vi "Get_file_list_table.vi"(10 "Filter pattern":string="*.xls", 11 "file path (dialog if empty)":path=path "C:/RIMAS/Temperature-logs") -> (0 "Files names":string[][](array[string]), 1 "selected path":path, 2 "Multicolumn Listbox":i32[](listbox), 3 "All Files in Dir":path[](array[path]))   [LabVIEW 2012]
panel:
  out "Array 2":dbl[](array[numeric])
  out "Justify arr":enum16{"Left", "Center", "Right"}[](array[ring])
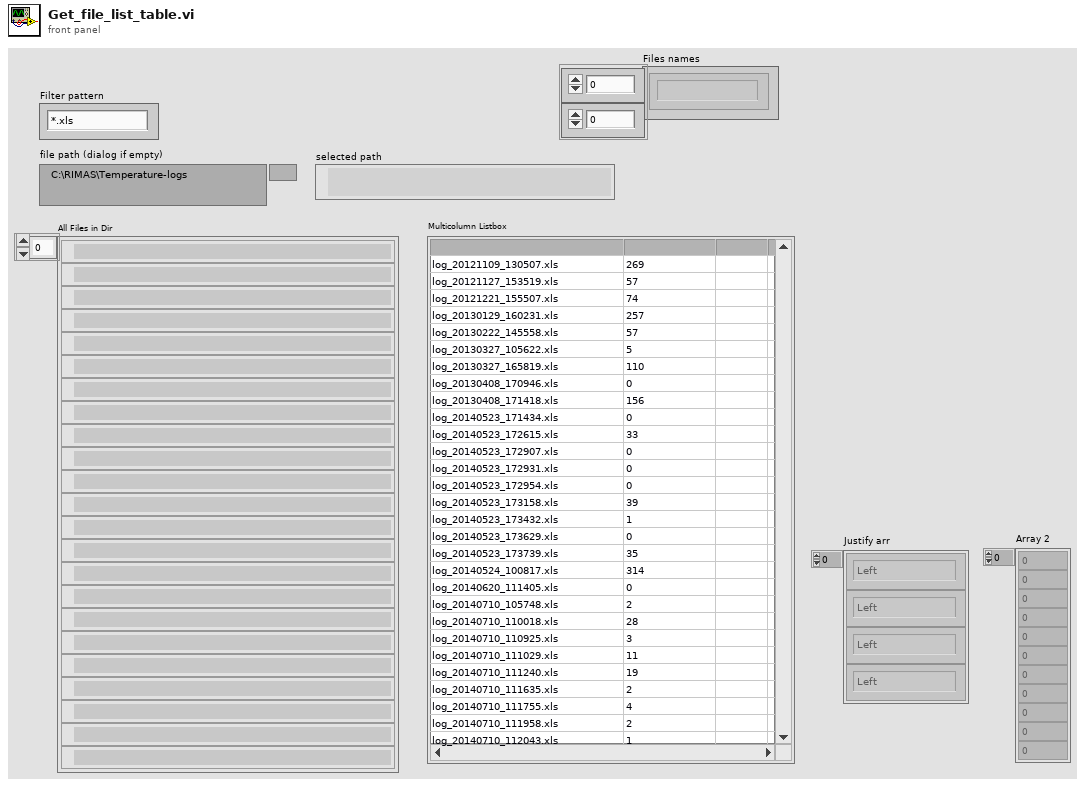
[diagram p1: front panel]
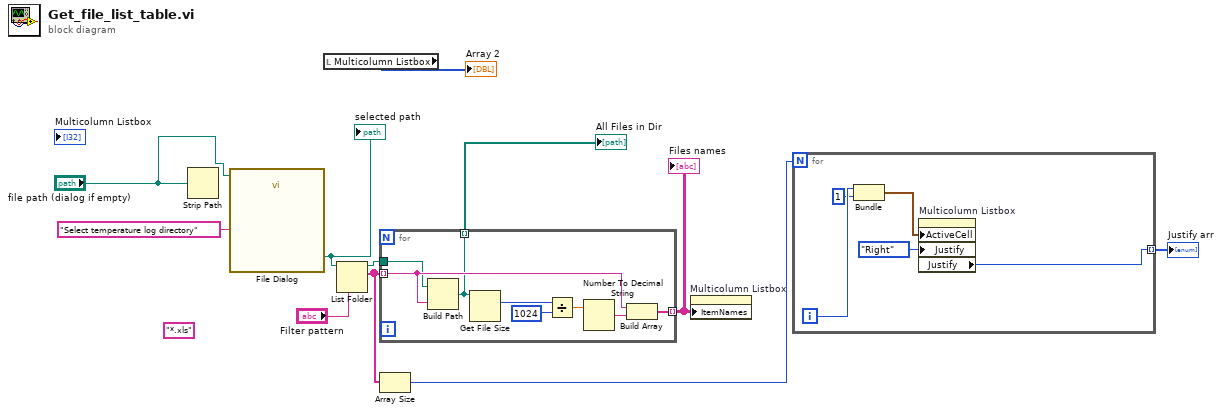
[diagram p0: block diagram]
diagram:
  (unwired) "*.xls" ("pattern (all files)")
  n1 = Strip Path(path="file path (dialog if empty)") -> ()  [unwired: 2 out]
  n2 = call "File Dialog"("start path"="file path (dialog if empty)", "prompt"="Select temperature log directory") -> ("selected path"=w11:path)  [unwired: 10 in, 3 out]
  "selected path" <- w11
  n3 = local read "Multicolumn Listbox"() -> (→"Array 2":i32[])
  n4 = List Folder(path=w11, pattern="Filter pattern") -> (path out=w6:path, filenames=w8:string[])  [unwired: 2 in, 2 out]
  n5 = for {
    tunnel: w8 -> [w17] mode=indexing
    tunnel: [w18] -> w10 mode=indexing
    tunnel: w6 -> [w16]
    tunnel: [w12] -> w5 mode=indexing
    n6 = Build Path(base path=w16, name or relative path=w17) -> (appended path=w12:path)
    n7 = Get File Size(file=w12) -> (size (in bytes)=w15:i64)  [unwired: 1 in, 2 out]
    n8 = Divide(x=w15, y=i64 1024) -> (x/y=w13:dbl)
    n9 = Number To Decimal String(number=w13) -> (decimal integer string=w19:string)  [unwired: 1 in]
    n10 = Build Array(w17, w19) -> (w18:string[])
  }
  "All Files in Dir" <- w5
  "Files names" <- w10
  n11 = Array Size(array=w8) -> (size(s)=w9:i32)
  n12 = property on="Multicolumn Listbox" class="MCListbox (strict)"("ItemNames"=w10) -> ()  [unwired: 2 in, 2 out]
  n13 = for {
    N: w9 -> [_]
    tunnel: [w21] -> w7 mode=indexing
    i -> [w23]
    n14 = Bundle(w23, "Column"=1) -> (w24:cluster{i32, "Column":i32})  [unwired: 1 in]
    n15 = property on="Multicolumn Listbox" class="MCListbox (strict)"("ActiveCell"=w24, "Justify"=enum16{"Left", "Center", "Right"}."Right" ("Active Cell:Cell Justification")) -> ("Justify"=w21:enum16{"Left", "Center", "Right"})  [unwired: 2 in, 2 out]
  }
  "Justify arr" <- w7
